vi "FPGA_AnalogTriggerConvertFPGAToSource.vi"(11 "FPGASourceType":T1) -> (3 "AnalogTriggerSource":T2={"Channel"=enum."AI 1", "Averaged"=FALSE, "Filter"=FALSE})   [LabVIEW 2017]
uses:
  <vilib>/Rock Robotics/SystemInterfaces/AnalogTrigger/FPGA_AnalogTriggerSource.ctl
  <vilib>/Rock Robotics/SystemInterfaces/AI/FPGA_AIChannel.ctl
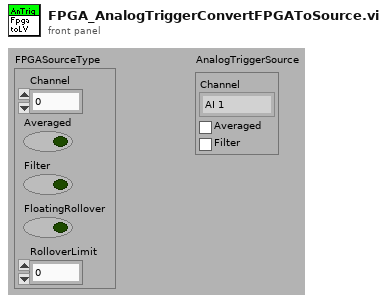
[diagram p1: front panel]
types:
  T1 = cluster{"Channel":fxp<+,3,3>, "Averaged":bool, "Filter":bool, "FloatingRollover":bool, "RolloverLimit":fxp<+/-,8,12>}
  T2 = typedef "FPGA_AnalogTriggerSource.ctl" = cluster{"Channel":T3, "Averaged":bool, "Filter":bool}
  T3 = typedef "FPGA_AIChannel.ctl" = enum8{"AI 0", "AI 1", "AI 2", "AI 3", "AI MXP 0", "AI MXP 1", "AI MXP 2", "AI MXP 3", "Invalid"}
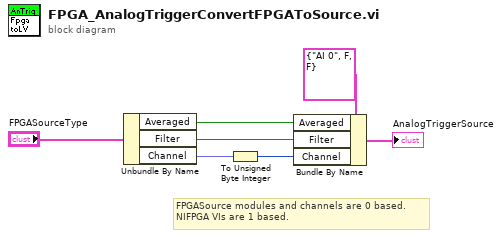
[diagram p0: block diagram]
diagram:
  # "FPGASource modules and channels are 0 based.\nNIFPGA VIs are 1 based."
  n1 = Unbundle By Name("FPGASourceType") -> ("Averaged"=w6:bool, "Filter"=w5:bool, "Channel"=w2:fxp<+,3,3>)
  n2 = To Unsigned Byte Integer(number=w2) -> (unsigned 8bit integer=w3:u8)
  n3 = Bundle By Name(cluster=T2 {"Channel"=enum."AI 0", "Averaged"=FALSE, "Filter"=FALSE} ("AnalogTriggerSource"), "Averaged"=w6, "Filter"=w5, "Channel"=w3) -> (→"AnalogTriggerSource":T2)
